vi "DSF.Engine.Transceiver Thread.Return to Thread Pool.vi"(8 "error in (no error)":errorcluster, 11 "Transceiver Thread in":refnum<class "DSF.Engine.Transceiver Thread.lvclass">) -> (0 "error out":errorcluster, 3 "Transceiver Thread out":refnum<class "DSF.Engine.Transceiver Thread.lvclass">)   [LabVIEW 2017, in "DSF.Engine.lvlib" / "DSF.Engine.Transceiver Thread.lvclass"]
uses:
  DSF.Engine.Transceiver Thread.lvclass
  DSF.Engine.Transceiver Thread.lvclass/DSF.Engine.Transceiver Thread.ctl
  Thread Parameters/Thread Parameters.lvclass/Thread Parameters.ctl
  Thread Pool/DSF.Engine.Pool.lvclass/DSF.Engine.Pool.ctl
  Debug/DSF.Engine.Debug Flags.FIFO.lvclass/DSF.Engine.Debug Flags.FIFO.ctl
  Thread Pool/DSF.Engine.Pool.Write FIFO.vi
  Thread Pool/DSF.Engine.Pool.Get FIFO.vi
  Thread Pool/DSF.Engine.Pool.Get Debug Flags.vi
  Debug/DSF.Engine.Debug Flags.FIFO.Get Infinite Timeouts.vi
  Thread Pool/DSF.Engine.Pool.ID.lvclass
  C:/github/data-sharing-framework/dsf core/Source/Engine/Classes/Thread Pool/DSF.Engine.Pool.lvclass
  Thread Parameters/Thread Parameters.lvclass
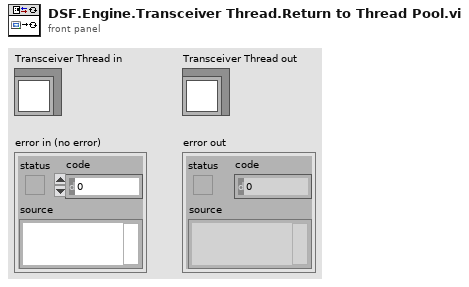
[diagram p1: front panel]
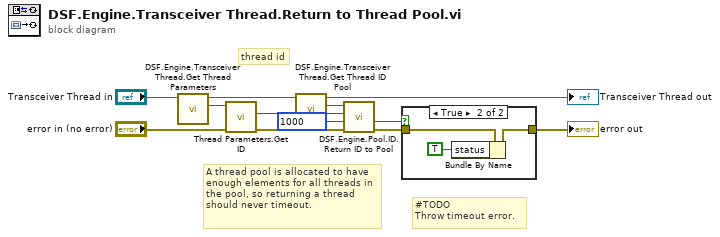
[diagram p0: block diagram]
diagram:
  # "thread id"
  # "A thread pool is allocated to have enough elements for all threads in the pool, so returning a thread should never timeout."
  # "#TODO\nThrow timeout error."
  n1 = call "DSF.Engine.Transceiver Thread.Get Thread Parameters.vi"("Transceiver Thread in"="Transceiver Thread in") -> ("Thread Parameters"=w4:refnum<class "Thread Parameters.lvclass">, "Transceiver Thread out"=w1:refnum<class "DSF.Engine.Transceiver Thread.lvclass">)  [unwired: 9 in]
  n2 = call "Thread Parameters.Get ID.vi"("Plugin in"=w4) -> ("id"=w3:i32)  [unwired: 9 in, 1 out]
  n3 = call "DSF.Engine.Transceiver Thread.Get Thread ID Pool.vi"("Transceiver Thread in"=w1) -> ("Thread ID Pool"=w11:refnum<class "DSF.Engine.Pool.ID.lvclass">, "Transceiver Thread out"=→"Transceiver Thread out":refnum<class "DSF.Engine.Transceiver Thread.lvclass">)  [unwired: 9 in]
  n4 = call "DSF.Engine.Pool.ID.Return ID to Pool.vi"("error in (no error)"="error in (no error)", "timeout in ms (0)"=1000, "id"=w3, "ID Pool in"=w11) -> ("error out"=w7:errorcluster, "timed out?"=w6:bool)  [unwired: 5 in, 1 out]
  n5 = case shown="True" w6 {
    tunnel: w7 -> [w12 w15]
    tunnel: [w12 w13] -> w5
    frame False {
    }
    frame True {
      n6 = Bundle By Name(cluster=w15, "status"=TRUE) -> (w13:errorcluster)
    }
  }
  "error out" <- w5
